vi "LED State Selector.vi"() -> ()   [LabVIEW 2016]
uses:
  LED Send Global.vi
panel:
  out "LED Message":string
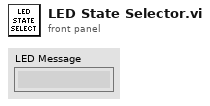
[diagram p1: front panel]
types:
  T1 = typedef "LED Send Global.ctl" = cluster{"Underglow States":cluster{"RED":bool, "BLUE":bool}, "Hopper States":cluster{"No Shooter Power":bool, "1 RED":bool, "2 RED":bool, "3 RED":bool, "1 YEL 3 RED":bool, "2 YEL 3 RED":bool, "3 YEL 3 RED":bool, "1 GRN 3 YEL 3 RED":bool, "2 GRN 3 YEL 3 RED":bool, "3 GRN 3 YEL 3 RED":bool, "All GRN":bool, "Shooter w/Agitator":bool}, "License Plate States":cluster{"Auton States":cluster{"Do Nothing":bool, "Gear":bool, "Gear & Baseline":bool, "Gear & Shooter":bool, "Shooter":bool, "Shooter & Ball Dump":bool}, "Drive Train":cluster{"High Gear":bool, "Low Gear":bool}}, "Misc":cluster{"Pit/Demo":bool}}
  T2 = cluster{"No Shooter Power":bool, "1 RED":bool, "2 RED":bool, "3 RED":bool, "1 YEL 3 RED":bool, "2 YEL 3 RED":bool, "3 YEL 3 RED":bool, "1 GRN 3 YEL 3 RED":bool, "2 GRN 3 YEL 3 RED":bool, "3 GRN 3 YEL 3 RED":bool, "All GRN":bool, "Shooter w/Agitator":bool}
  T3 = cluster{"Do Nothing":bool, "Gear":bool, "Gear & Baseline":bool, "Gear & Shooter":bool, "Shooter":bool, "Shooter & Ball Dump":bool}
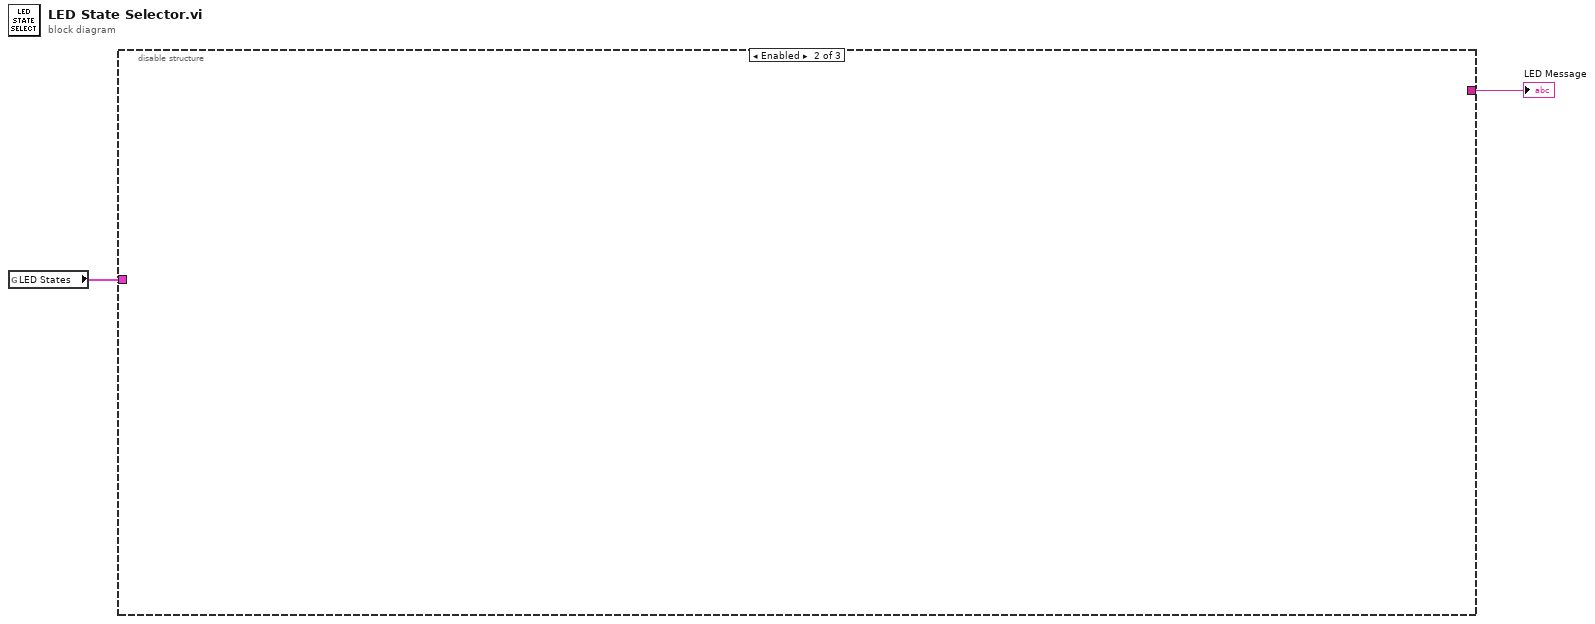
[diagram p0: block diagram]
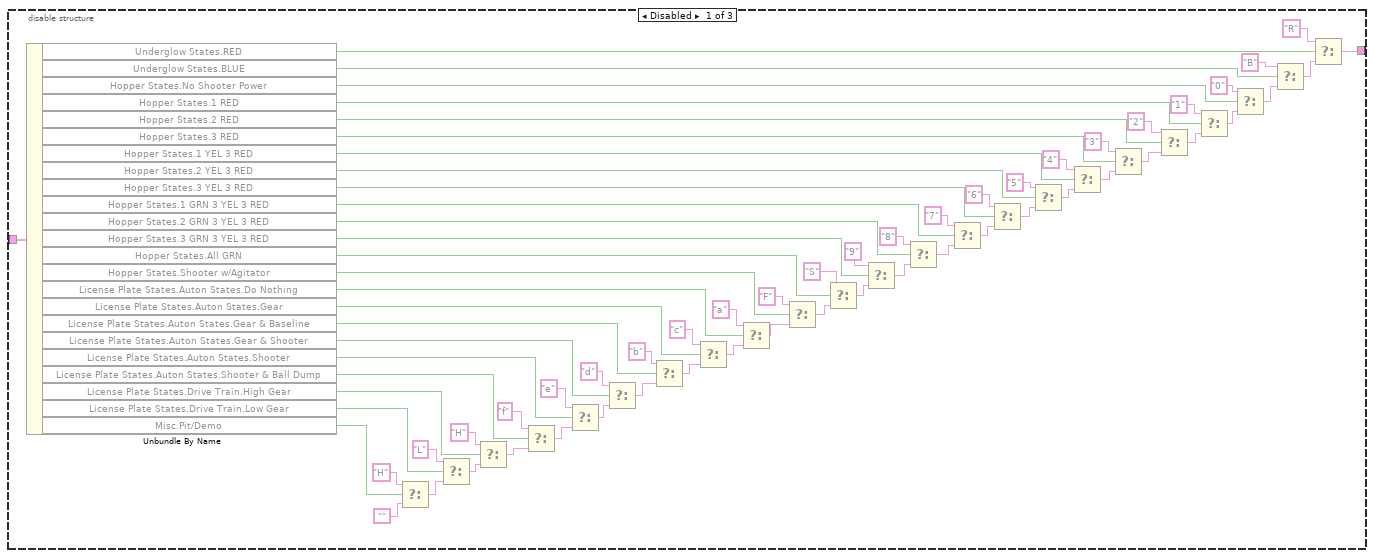
[diagram p2: hidden frame]
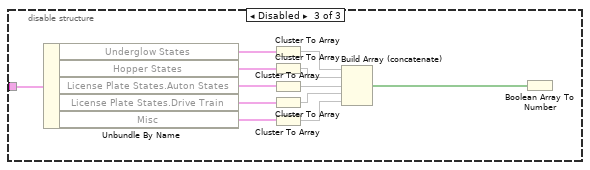
[diagram p3: hidden frame]
diagram:
  n1 = global read "LED Send Global.vi" "LED States"() -> (w2:T1)
  n2 = disable-structure shown="Enabled" {
    disable-tunnel: w2 -> [w73 _ w85]
    disable-tunnel: [w28 _ _] -> w1
    frame Disabled {
      n3 = Unbundle By Name(w73) -> ("Underglow States.RED"=w72:bool, "Underglow States.BLUE"=w69:bool, "Hopper States.No Shooter Power"=w66:bool, "Hopper States.1 RED"=w62:bool, "Hopper States.2 RED"=w60:bool, "Hopper States.3 RED"=w57:bool, "Hopper States.1 YEL 3 RED"=w53:bool, "Hopper States.2 YEL 3 RED"=w50:bool, "Hopper States.3 YEL 3 RED"=w47:bool, "Hopper States.1 GRN 3 YEL 3 RED"=w44:bool, "Hopper States.2 GRN 3 YEL 3 RED"=w42:bool, "Hopper States.3 GRN 3 YEL 3 RED"=w38:bool, "Hopper States.All GRN"=w36:bool, "Hopper States.Shooter w/Agitator"=w32:bool, "License Plate States.Auton States.Do Nothing"=w29:bool, "License Plate States.Auton States.Gear"=w26:bool, "License Plate States.Auton States.Gear & Baseline"=w22:bool, "License Plate States.Auton States.Gear & Shooter"=w19:bool, "License Plate States.Auton States.Shooter"=w17:bool, "License Plate States.Auton States.Shooter & Ball Dump"=w13:bool, "License Plate States.Drive Train.High Gear"=w10:bool, "License Plate States.Drive Train.Low Gear"=w7:bool, "Misc.Pit/Demo"=w4:bool)
      n4 = Select(t="H", s=w4, f="") -> (s? t:f=w6:string)
      n5 = Select(t="L", s=w7, f=w6) -> (s? t:f=w9:string)
      n6 = Select(t="H", s=w10, f=w9) -> (s? t:f=w11:string)
      n7 = Select(t="f", s=w13, f=w11) -> (s? t:f=w15:string)
      n8 = Select(t="e", s=w17, f=w15) -> (s? t:f=w18:string)
      n9 = Select(t="d", s=w19, f=w18) -> (s? t:f=w21:string)
      n10 = Select(t="b", s=w22, f=w21) -> (s? t:f=w24:string)
      n11 = Select(t="c", s=w26, f=w24) -> (s? t:f=w27:string)
      n12 = Select(t="a", s=w29, f=w27) -> (s? t:f=w31:string)
      n13 = Select(t="F", s=w32, f=w31) -> (s? t:f=w34:string)
      n14 = Select(t="S", s=w36, f=w34) -> (s? t:f=w37:string)
      n15 = Select(t="9", s=w38, f=w37) -> (s? t:f=w40:string)
      n16 = Select(t="8", s=w42, f=w40) -> (s? t:f=w43:string)
      n17 = Select(t="7", s=w44, f=w43) -> (s? t:f=w46:string)
      n18 = Select(t="6", s=w47, f=w46) -> (s? t:f=w49:string)
      n19 = Select(t="5", s=w50, f=w49) -> (s? t:f=w52:string)
      n20 = Select(t="4", s=w53, f=w52) -> (s? t:f=w55:string)
      n21 = Select(t="3", s=w57, f=w55) -> (s? t:f=w58:string)
      n22 = Select(t="2", s=w60, f=w58) -> (s? t:f=w61:string)
      n23 = Select(t="1", s=w62, f=w61) -> (s? t:f=w64:string)
      n24 = Select(t="0", s=w66, f=w64) -> (s? t:f=w67:string)
      n25 = Select(t="B", s=w69, f=w67) -> (s? t:f=w70:string)
      n26 = Select(t="R", s=w72, f=w70) -> (s? t:f=w28:string)
    }
    frame Enabled {
    }
    frame Disabled {
      n27 = Unbundle By Name(w85) -> ("Underglow States"=w84:cluster{"RED":bool, "BLUE":bool}, "Hopper States"=w83:T2, "License Plate States.Auton States"=w82:T3, "License Plate States.Drive Train"=w81:cluster{"High Gear":bool, "Low Gear":bool}, "Misc"=w80:cluster{"Pit/Demo":bool})
      n28 = Cluster To Array(cluster=w84) -> (array=w75:bool[])
      n29 = Cluster To Array(cluster=w83) -> (array=w79:bool[])
      n30 = Cluster To Array(cluster=w82) -> (array=w78:bool[])
      n31 = Cluster To Array(cluster=w81) -> (array=w77:bool[])
      n32 = Cluster To Array(cluster=w80) -> (array=w76:bool[])
      n33 = Build Array (concatenate)(w75, w79, w78, w77, w76) -> (w74:bool[])
      n34 = Boolean Array To Number(Boolean array=w74) -> ()  [unwired: 1 out]
    }
  }
  "LED Message" <- w1
